vi "Voltage - HW-Timed Single Point Input.vi"() -> ()   [LabVIEW 2022 SP3]
doc: "This example demonstrates how to continuously acquire voltage measurements from a DAQmx device using hardware timed, single point reads. This means that for each loop iteration, a single sample is read from the device. The device will read data on each tick of the sample clock. If an additional sample clock tick occurs before the current data point is read from the device, an error will be thrown indicating that this has happened. To ignore these errors, set the \"Convert Late Errors To Warnings\" control to TRUE.\n\nHardware Timed Single Point acquisition works best when using a deterministic operating system (such as LabVIEW Real-Time). Because of the less deterministic nature of general purpose operating systems (such as Microsoft Windows), the software loop will not always take the exact same amount of time to execute, and this may lead to the occasional missed sample clock. If missed sample clock errors become an issue, you can try decreasing the sample rate, or setting the \"Convert Late Errors To Warnings\" control to TRUE.\n\nFor instructions on how to connect your signals to the DAQ device, refer to your device documentation."
uses:
  <vilib>/Utility/error.llb/DialogType.ctl
  <vilib>/DAQmx/read.llb/DAQmx Read (Analog 1D DBL NChan 1Samp).vi
  <vilib>/DAQmx/create/channels.llb/DAQmx Create Channel (AI-Voltage-Basic).vi
  <vilib>/DAQmx/configure/timing.llb/DAQmx Timing (Sample Clock).vi
  <vilib>/DAQmx/miscellaneous.llb/DAQmx Fill In Error Info.vi
  <resource>/objmgr/daqmx.rc
panel:
  in  "Convert Late Errors to Warnings?":bool
  in  "Stop":bool
  out "Waveform Chart":dbl[][](graph)
  in  "Sample Rate":dbl=100.0
  in  "Sample Clock Source":tag="OnboardClock"
  in  "Terminal Configuration":i32(ring)=-1 items=["default"=-1, "RSE"=10083, "NRSE"=10078, "Differential"=10106, "Pseudodifferential"=12529]
  in  "Max Voltage":dbl=5.0
  in  "Min Voltage":dbl=-5.0
  in  "Physical Channel":tag="Dev1/ai0"
  out "Actual Sample Rate":dbl=100.0 format="%0.2f"
  # "Channel Settings"
  # "Acquired Data"
  # "Timing Settings"
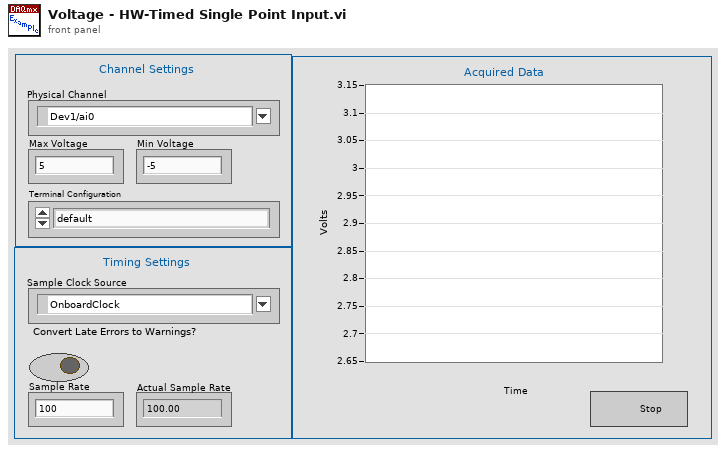
[diagram p1: front panel]
types:
  T1 = typedef "DialogType.ctl" = u16
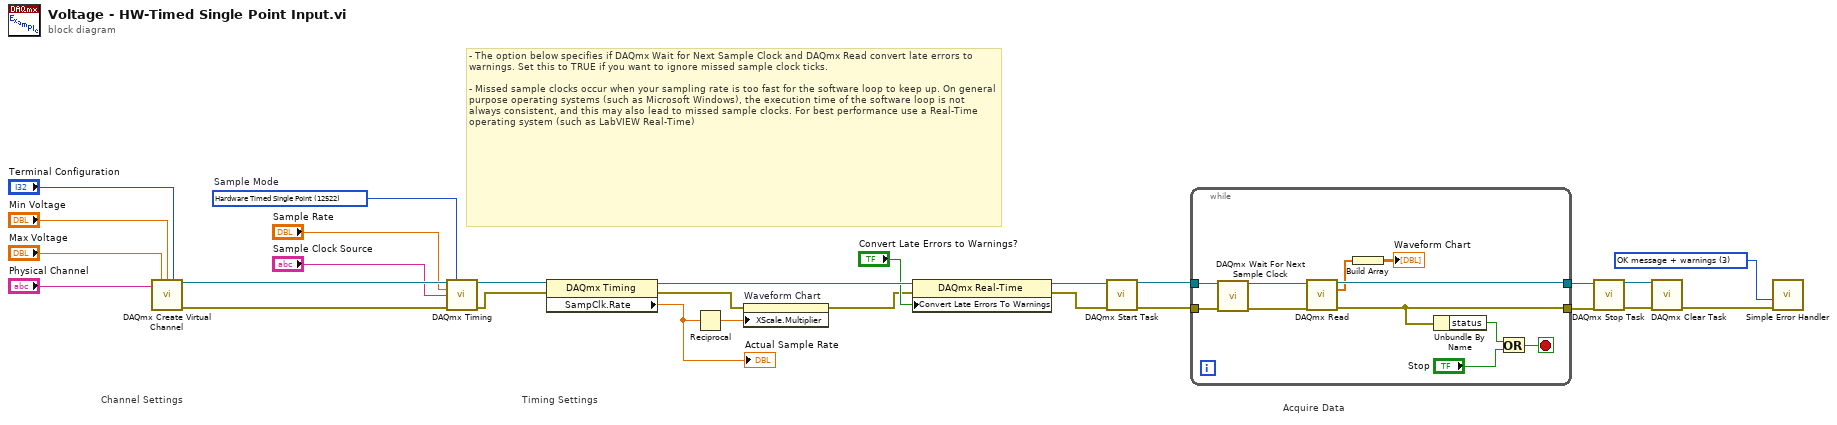
[diagram p0: block diagram]
diagram:
  w6 = T1 3 items=["no dialog", "OK message", "continue or stop message", "OK message + warnings", "continue/stop + warnings"] ("type of dialog (OK msg:1)")
  w25 = 12522 items=["Finite Samples"=10178, "Continuous Samples"=10123, "Hardware Timed Single Point"=12522]  # Sample Mode
  # "- The option below specifies if DAQmx Wait for Next Sample Clock and DAQmx Read convert late errors to warnings. Set this to TRUE if you want to ignore missed sample clock ticks.\n \n- Missed sample clocks occur when your sampling rate is too fast for the software loop to keep up. On general purpose operating systems (such as Microsoft Windows), the execution time of the software loop is not always consistent, and this may also lead to missed sample clocks. For best performance use a Real-Time operating system (such as LabVIEW Real-Time)"
  # "Acquire Data"
  # "Timing Settings"
  # "Channel Settings"
  n1 = call-poly <vilib>:"DAQmx Create Virtual Channel.vi"("maximum value"="Max Voltage", "minimum value"="Min Voltage", "input terminal configuration"="Terminal Configuration", "physical channels"="Physical Channel") -> ("task out"=w23:refnum<k21>, "error out"=w24:errorcluster)  [unwired: 10 in]
  n2 = call-poly <vilib>:"DAQmx Timing.vi"("task/channels in"=w23, "sample mode"=w25, "rate"="Sample Rate", "source"="Sample Clock Source", "error in"=w24) -> ("task out"=w27:refnum<k21>, "error out"=w26:errorcluster)  [unwired: 9 in]
  n3 = property class="DAQmx Timing"(reference=w27, error in=w26) -> (reference out=w9:refnum<k21>, error out=w2:errorcluster, "SampClk.Rate"=w4:dbl)
  "Actual Sample Rate" <- w4
  n4 = Reciprocal(x=w4) -> (1/x=w5:dbl)
  n5 = property on="Waveform Chart" class="WFChart (strict)"(error in=w2, "XScale.Multiplier"=w5) -> (error out=w3:errorcluster)  [unwired: 1 in, 1 out]
  n6 = property class="DAQmx Real-Time"(reference=w9, error in=w3, "Convert Late Errors To Warnings"="Convert Late Errors to Warnings?") -> (reference out=w8:refnum<k21>, error out=w1:errorcluster)
  n7 = call <vilib>:"DAQmx Start Task.vi"("task/channels in"=w8, "error in"=w1) -> ("task out"=w22:refnum<k21>, "error out"=w21:errorcluster)  [unwired: 12 in]
  n8 = while {
    tunnel: w22 -> [w31]
    tunnel: w21 -> [w38]
    tunnel: [w34] -> w13
    tunnel: [w33] -> w12
    stop <- w35 stop-if-true
    n9 = call <vilib>:"DAQmx Wait For Next Sample Clock.vi"("task/channels in"=w31, "error in"=w38) -> ("task out"=w30:refnum<k21>, "error out"=w32:errorcluster)  [unwired: 11 in, 1 out]
    n10 = call-poly <vilib>:"DAQmx Read.vi"("task/channels in"=w30, "error in"=w32) -> ("task out"=w34:refnum<k21>, "data"=w29:dbl[], "error out"=w33:errorcluster)  [unwired: 11 in]
    n11 = Build Array(w29) -> (→"Waveform Chart":dbl[][])
    n12 = Unbundle By Name(w33) -> ("status"=w36:bool)
    n13 = Or(x=w36, y="Stop") -> (x .or. y?=w35:bool)
  }
  n14 = call <vilib>:"DAQmx Stop Task.vi"("task/channels in"=w13, "error in"=w12) -> ("task out"=w10:refnum<k21>, "error out"=w11:errorcluster)  [unwired: 12 in]
  n15 = call <vilib>:"DAQmx Clear Task.vi"("task in"=w10, "error in"=w11) -> ("error out"=w20:errorcluster)  [unwired: 13 in]
  n16 = call <vilib>:"Simple Error Handler.vi"("type of dialog (OK msg:1)"=w6, "error in (no error)"=w20) -> ()  [unwired: 3 in, 5 out]
